vi "Synchronize to RT (FPGA) - cRIO.vi"() -> ()   [LabVIEW 2010]
uses:
  <vilib>/Platform/TimedLoop/XDataNode/XDataNode.xnode
  <vilib>/Platform/TimedLoop/XDataNode/timing_clust.ctl
  <vilib>/Platform/TimedLoop/XDataNode/nitl_modes.ctl
  <vilib>/Platform/TimedLoop/XDataNode/wakeup.ctl
  FPGA Timekeeper.lvlib
  <vilib>/Platform/TimedLoop/XDataNode/XDNodeRunTimeDep.lvlib
panel:
  in  "RT time (ns)":u64
  out "offset from RT time (ns)":i32
  out "FPGA Timekeeper locked":bool
  out "FPGA Timekeeper time (ns)":u64
  # "This example synchronizes the FPGA Timekeeper on a CompactRIO FPGA target with the current system time of a Real-Time target."
  # "FPGA Timekeeper"
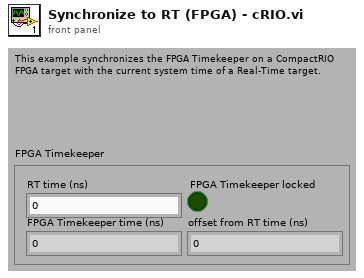
[diagram p1: front panel]
types:
  T1 = typedef "XDNodeRunTimeDep.lvlib/timing_clust.ctl" = cluster{"Expected End [f-1]":u64, "Actual End [f-1]":u64, "Finished Late? [f-1]":bool, "Expected End [i-1]":u64, "Actual End [i-1]":u64, "Finished Late? [i-1]":bool, "Expected Start [i]":u64, "Actual Start [i]":u64, "Expected Start [f]":u64, "Actual Start [f]":u64, "Source Name":string, "Structure Name":string, "Period":i64, "Deadline":i64, "Offset":i64, "Start":i64, "Priority":i32, "Timeout":i32, "Mode":T2, "Wakeup Reason":T3, "Error":errorcluster, "Source Type":string, "Secondary Source Type":string, "Global End Time":u64, "Global Start Time":u64, "Frame Duration":u64, "Iteration Duration":u64, "Assigned CPU":i32, "I/O Scan Engine Mode":u32}
  T2 = typedef "XDNodeRunTimeDep.lvlib/nitl_modes.ctl" = enum32{"No Change", "Process missed periods, maintain original phase", "Discard missed periods, maintain original phase", "Process missed periods, ignore original phase", "Discard missed periods, ignore original phase"}
  T3 = typedef "XDNodeRunTimeDep.lvlib/wakeup.ctl" = enum32{"Normal", "Aborted", "Asynchronous wakeup", "Timing source error", "Timed loop error", "Timeout"}
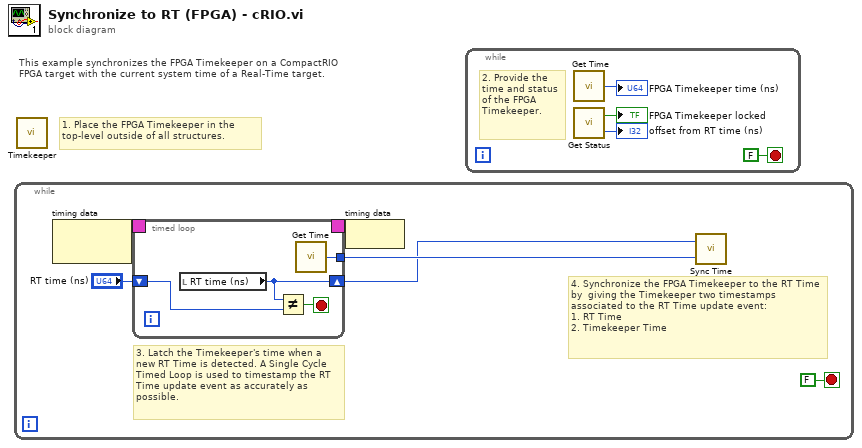
[diagram p0: block diagram]
diagram:
  # "This example synchronizes the FPGA Timekeeper on a CompactRIO FPGA target with the current system time of a Real-Time target."
  # "1. Place the FPGA Timekeeper in the top-level outside of all structures."
  n1 = while {
    stop <- FALSE stop-if-true
    # "3. Latch the Timekeeper's time when a new RT Time is detected. A Single Cycle Timed Loop is used to timestamp the RT Time update event as accurately as possible."
    # "4. Synchronize the FPGA Timekeeper to the RT Time by  giving the Timekeeper two timestamps associated to the RT Time update event:\n1. RT Time\n2. Timekeeper Time"
    n2 = node-c288() -> (w6:T1)  [unwired: 1 in]
    n3 = timed-loop {
      timing: w6 -> [_]
      timing-out: [_] -> w5
      shift-right: [w7] -> w1
      shift-left: "RT time (ns)" -> [w8]
      tunnel: [w10] -> w4
      stop <- w9 stop-if-true
      n4 = local read "RT time (ns)"() -> (w7:u64)
      n5 = Not Equal?(x=w7, y=w8) -> (x != y?=w9:bool)
      n6 = call "Get Time.vi"() -> ("time (ns)"=w10:u64)
    }
    n7 = node-c288(w5) -> ()
    n8 = call "Sync Time.vi"("FPGA Timekeeper time (ns)"=w4, "time reference time (ns)"=w1) -> ()
  }
  n9 = call "Timekeeper.vi"() -> ()  [unwired: 12 in]
  n10 = while {
    stop <- FALSE stop-if-true
    # "2. Provide the time and status of the FPGA Timekeeper."
    n11 = call "Get Time.vi"() -> ("time (ns)"=→"FPGA Timekeeper time (ns)":u64)
    n12 = call "Get Status.vi"() -> ("FPGA Timekeeper locked"=→"FPGA Timekeeper locked":bool, "offset from time reference"=→"offset from RT time (ns)":i32)
  }
